vi "sequencer.vi"() -> ()   [LabVIEW 2020]
uses:
  <vilib>/Utility/file.llb/Read Delimited Spreadsheet (string).vi
panel:
  out "String 4":string
  out "String 3":string
  out "String 2":string
  out "String":string
  in  "stop":bool
  in  "Time per measurement":u32
  in  "File path (dialog if empty)":path
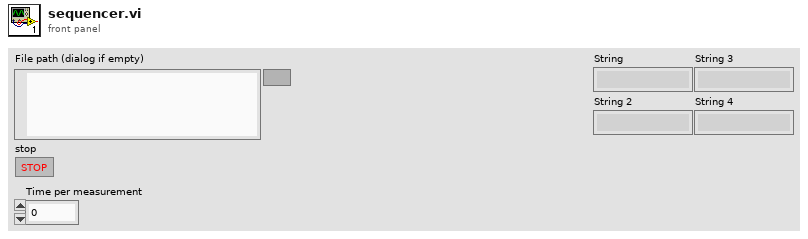
[diagram p1: front panel]
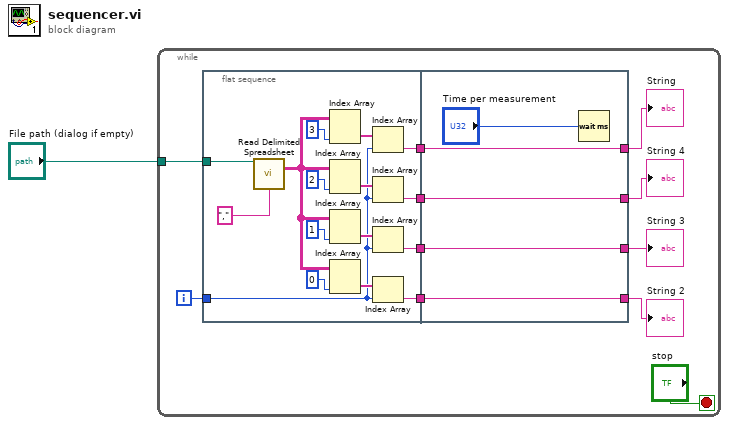
[diagram p0: block diagram]
diagram:
  n1 = while {
    tunnel: "File path (dialog if empty)" -> [w8]
    i -> [w7]
    stop <- "stop" stop-if-true
    n2 = flat-sequence {
      tunnel: w8 -> [w28]
      tunnel: [w18] -> w12
      tunnel: [w17] -> w11
      tunnel: [w16] -> w10
      tunnel: [w15] -> w9
      tunnel: w7 -> [w14]
      tunnel: w12 -> [w32]
      tunnel: [w32] -> w2
      tunnel: w11 -> [w31]
      tunnel: [w31] -> w4
      tunnel: w10 -> [w30]
      tunnel: [w30] -> w3
      tunnel: w9 -> [w29]
      tunnel: [w29] -> w5
      frame #0 {
        n3 = call-poly <vilib>:"Read Delimited Spreadsheet.vi"("file path (dialog if empty)"=w28, "delimiter (\\t)"="," ("delimiter (\\t)")) -> ("all rows"=w23:string[][])  [unwired: 8 in, 5 out]
        n4 = Index Array(array=w23, index (col)=3) -> (element=w19:string[])  [unwired: 1 in]
        n5 = Index Array(array=w23, index (col)=2) -> (element=w20:string[])  [unwired: 1 in]
        n6 = Index Array(array=w23, index (col)=1) -> (element=w21:string[])  [unwired: 1 in]
        n7 = Index Array(array=w23, index (col)=0) -> (element=w22:string[])  [unwired: 1 in]
        n8 = Index Array(array=w19, index=w14) -> (element=w15:string)
        n9 = Index Array(array=w20, index=w14) -> (element=w16:string)
        n10 = Index Array(array=w21, index=w14) -> (element=w17:string)
        n11 = Index Array(array=w22, index=w14) -> (element=w18:string)
      }
      frame #1 {
        n12 = Wait (ms)(milliseconds to wait="Time per measurement") -> ()  [unwired: 1 out]
      }
    }
    "String" <- w5
    "String 3" <- w4
    "String 4" <- w3
    "String 2" <- w2
  }
